vi "Units_MetersToFeet.vi"(10 "Meters":dbl) -> (2 "Feet":dbl)   [LabVIEW 2019, in "Trajectory_Library.lvlib"]
doc: "Convert a value from meters to feet\n\nInputs: \n - Meters - Distance (Meters)\n\nOutputs:\n - Feet - Distance (Feet)"
uses:
  Trajectory_Library.lvlib
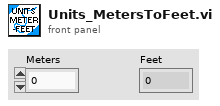
[diagram p1: front panel]
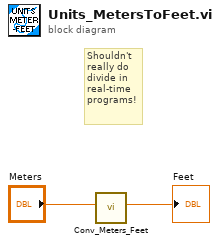
[diagram p0: block diagram]
diagram:
  # "Shouldn't\nreally do\ndivide in\nreal-time\nprograms!"
  n1 = call "Conv_Meters_Feet.vi"("Meters"="Meters") -> ("Feet"=→"Feet":dbl)  [unwired: 10 in]
